vi "MoveMultipleJogSteps.vi"(8 "Error In":errorcluster, 9 "Step Amounts":dbl, 10 "direction":i32(ring)=1 items=["Forward"=1, "Backward"=2], 11 "Thorlabs In":refnum<class "Thorlabs.lvclass">) -> (0 "Error Out":errorcluster, 3 "Thorlabs Out":refnum<class "Thorlabs.lvclass">)   [LabVIEW 2018, in "Thorlabs.lvlib" / "Thorlabs.lvclass"]
doc: "Moves the Axis by a the step size for the job parameters. This is done in the direction specified.\n\nCreator: Slade Jeppesen\nCreated Date: 10/02/20"
uses:
  Thorlabs.lvclass
  Thorlabs.lvclass/Thorlabs.ctl
  C:/AME Test Engineering/LabVIEW/PPLs/Axis/DLLs/ThorLabs.MotionControl.KCube.DCServoCLI.dll
  PPLs/Axis/DLLs/ThorLabs.MotionControl.KCube.DCServoCLI.dll
  31825a4c-c9b7-413c-8d5f-0f6836adbe55.vi
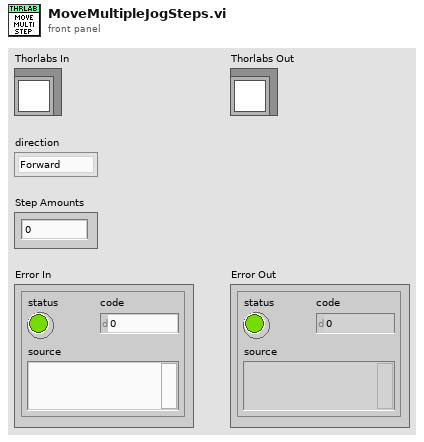
[diagram p1: front panel]
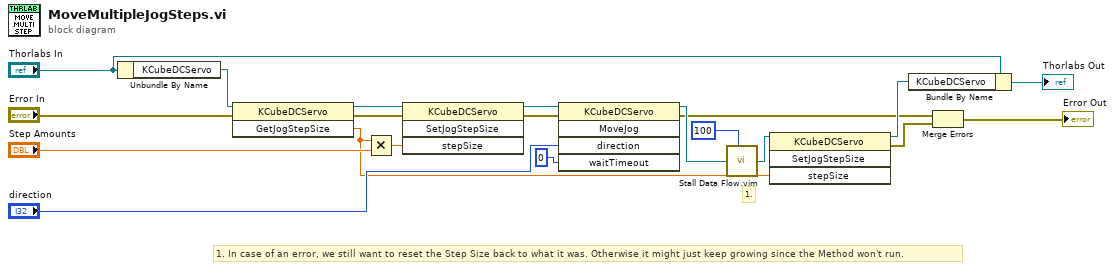
[diagram p0: block diagram]
diagram:
  # "1. In case of an error, we still want to reset the Step Size back to what it was. Otherwise it might just keep growing since the Method won't run."
  # "1."
  n1 = Unbundle By Name("Thorlabs In") -> ("KCubeDCServo"=w15:refnum<k24>)
  n2 = invoke class="KCubeDCServo" method="GetJogStepSize"(reference=w15, error in="Error In") -> (reference out=w12:refnum<k24>, error out=w11:errorcluster, "GetJogStepSize"=w6:dbl)  [unwired: 1 in]
  n3 = Multiply(x=w6, y="Step Amounts") -> (x*y=w13:dbl)
  n4 = invoke class="KCubeDCServo" method="SetJogStepSize"(reference=w12, error in=w11, "stepSize"=w13) -> (reference out=w8:refnum<k24>, error out=w9:errorcluster)  [unwired: 1 in, 2 out]
  n5 = invoke class="KCubeDCServo" method="MoveJog"(reference=w8, error in=w9, "direction"="direction", "waitTimeout"=0) -> (reference out=w5:refnum<k24>, error out=w2:errorcluster)  [unwired: 1 in, 3 out]
  n6 = call "Stall Data Flow.vim"("value in"=w5, "milliseconds to wait"=u32 100) -> ("value out"=w4:refnum<k24>)  [unwired: 1 out]
  n7 = invoke class="KCubeDCServo" method="SetJogStepSize"(reference=w4, "stepSize"=w6) -> (reference out=w7:refnum<k24>, error out=w3:errorcluster)  [unwired: 2 in, 2 out]
  n8 = Bundle By Name(cluster="Thorlabs In", "KCubeDCServo"=w7) -> (→"Thorlabs Out":refnum<class "Thorlabs.lvclass">)
  n9 = Merge Errors(w2, w3) -> (→"Error Out":errorcluster)
